vi "Send CSI.vi"(8 "csi valid":bool=TRUE, 9 "channel estimate timing":T2, 10 "channel estimate":T1, 11 "format":enum16{"NON_HT_OFDM", "VHT", "NON_HT_DUP_OFDM"}(ring)) -> ()   [LabVIEW 2020]
uses:
  <vilib>/rvi/interface/RandomDataEmulation/niFpgaRandomDataHandleErrors.vi
  <vilib>/rvi/DataTransferAndStorage/Container/XNode/niFpgaContainer.xnode
  <vilib>/rvi/interface/RandomDataEmulation/nirviRandomDataFpgaReadWriteTemplate.vi
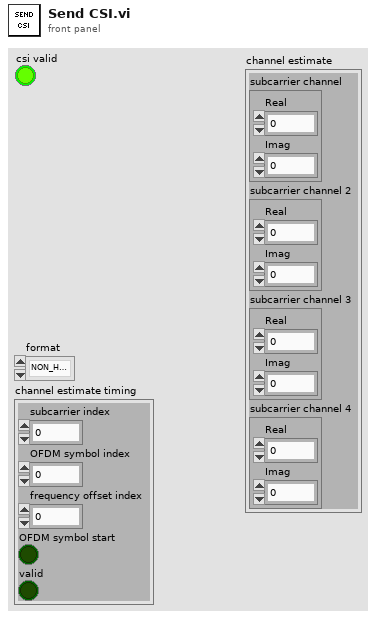
[diagram p1: front panel]
types:
  T1 = cluster{"subcarrier channel":cluster{"Real":fxp<+/-,25,4>, "Imag":fxp<+/-,25,4>}, "subcarrier channel 2":cluster{"Real":fxp<+/-,25,4>, "Imag":fxp<+/-,25,4>}, "subcarrier channel 3":cluster{"Real":fxp<+/-,25,4>, "Imag":fxp<+/-,25,4>}, "subcarrier channel 4":cluster{"Real":fxp<+/-,25,4>, "Imag":fxp<+/-,25,4>}}
  T2 = cluster{"subcarrier index":u8, "OFDM symbol index":u16, "frequency offset index":fxp<+/-,9,9>, "OFDM symbol start":bool, "valid":bool}
  T3 = cluster{"Real":fxp<+/-,25,4>, "Imag":fxp<+/-,25,4>}
  T4 = cluster{"L-STF-1":bool, "L-STF-2":bool, "L-LTF-1":bool, "L-LTF-2":bool, "L-SIG":bool, "VHT-Data":bool, "VHT-Data Init":bool, "VHT-SIG-B":bool, "VHT-LTF":bool, "VHT-STF":bool, "VHT-SIG A-2":bool, "VHT-SIG A-1":bool, "L-Data":bool, "L-Data Init":bool}
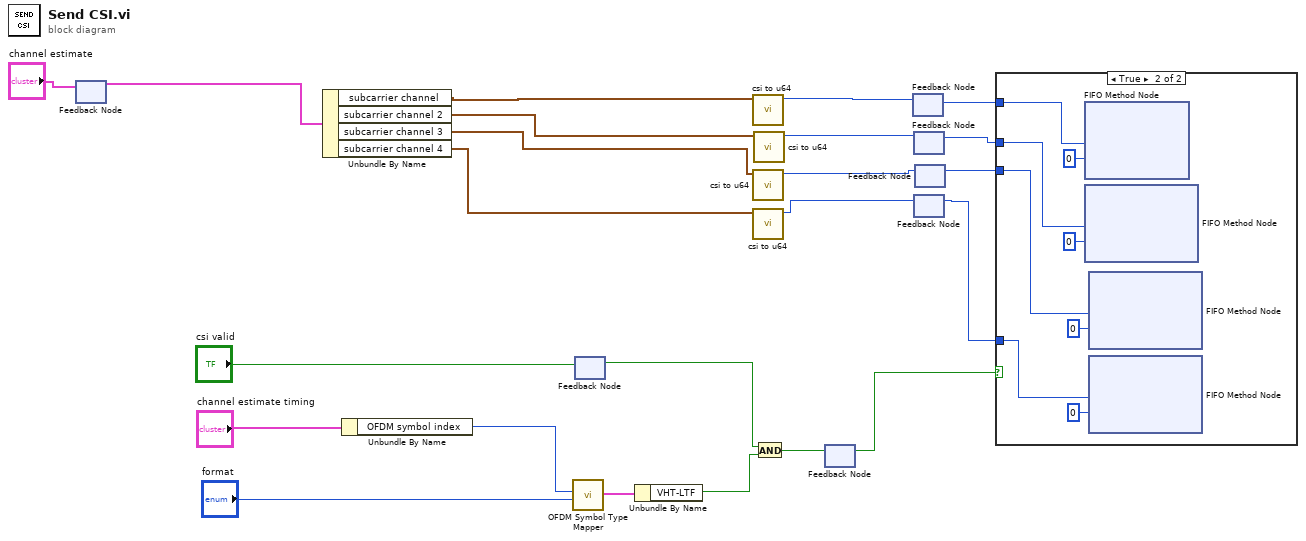
[diagram p0: block diagram]
diagram:
  n1 = feedback #1() -> (w1:T1)  [unwired: 1 in]
  n2 = feedback-in #1("channel estimate") -> ()
  n3 = Unbundle By Name(w1) -> ("subcarrier channel"=w11:T3, "subcarrier channel 2"=w10:T3, "subcarrier channel 3"=w9:T3, "subcarrier channel 4"=w8:T3)
  n4 = Unbundle By Name("channel estimate timing") -> ("OFDM symbol index"=w21:u16)
  n5 = call "OFDM Symbol Type Mapper.vi"("format"="format", "OFDM symbol index"=w21) -> ("Cluster"=w20:T4)  [unwired: 9 in]
  n6 = feedback-in #2("csi valid") -> ()
  n7 = feedback #2() -> (w19:bool)  [unwired: 1 in]
  n8 = Unbundle By Name(w20) -> ("VHT-LTF"=w13:bool)
  n9 = call "csi to u64.vi"("subcarrier channel"=w11) -> ("Numeric"=w15:u64)  [unwired: 10 in]
  n10 = call "csi to u64.vi"("subcarrier channel"=w9) -> ("Numeric"=w6:u64)  [unwired: 10 in]
  n11 = call "csi to u64.vi"("subcarrier channel"=w8) -> ("Numeric"=w5:u64)  [unwired: 10 in]
  n12 = call "csi to u64.vi"("subcarrier channel"=w10) -> ("Numeric"=w7:u64)  [unwired: 10 in]
  n13 = And(x=w19, y=w13) -> (x .and. y?=w18:bool)
  n14 = feedback #3() -> (w17:bool)  [unwired: 1 in]
  n15 = feedback-in #3(w18) -> ()
  n16 = feedback #4() -> (w16:u64)  [unwired: 1 in]
  n17 = feedback-in #4(w15) -> ()
  n18 = feedback #5() -> (w4:u64)  [unwired: 1 in]
  n19 = feedback-in #5(w7) -> ()
  n20 = feedback #6() -> (w2:u64)  [unwired: 1 in]
  n21 = feedback-in #6(w5) -> ()
  n22 = feedback #7() -> (w3:u64)  [unwired: 1 in]
  n23 = feedback-in #7(w6) -> ()
  n24 = case shown="True" w17 {
    tunnel: w16 -> [_ w30]
    tunnel: w4 -> [_ w26]
    tunnel: w3 -> [_ w25]
    tunnel: w2 -> [_ w24]
    frame False {
    }
    frame True {
      n25 = xnode ("FIFO Method Node")("Element"=w30, "Timeout"=0) -> ()  [unwired: 1 in, 2 out]
      n26 = xnode ("FIFO Method Node")("Element"=w26, "Timeout"=0) -> ()  [unwired: 1 in, 2 out]
      n27 = xnode ("FIFO Method Node")("Element"=w25, "Timeout"=0) -> ()  [unwired: 1 in, 2 out]
      n28 = xnode ("FIFO Method Node")("Element"=w24, "Timeout"=0) -> ()  [unwired: 1 in, 2 out]
    }
  }
